vi "_DSF file channels to data.vi"(8 "error in (no error)":errorcluster, 10 "transfer":T7, 11 "configuration file cluster in":T1) -> (0 "error out":errorcluster, 2 "channels":T13[](array[typedef]), 3 "configuration file cluster out":T1)   [LabVIEW 2017, in "DSF Configuration API v1.0.0.lvlib"]
uses:
  DSF Configuration API v1.0.0.lvlib
  Controls/dsf configuration data/1.0.0/dsf settings.ctl
  Controls/dsf configuration data/1.0.0/dsf configuration data v1.0.0.lvlib
  Controls/dsf configuration data/1.0.0/dsf channel.ctl
  get item value by id/get channel value by id.vi
  get item value by id/get setting value by id.vi
  Controls/dsf configuration file/1.0.0/DSF Transfer.ctl
  File API/DSFConfig.lvlib
  Controls/dsf configuration file/1.0.0/DSF Channel.ctl
  Controls/dsf configuration file/1.0.0/dsf timing.ctl
  Controls/dsf configuration file/1.0.0/DSF Group.ctl
  Controls/dsf configuration file/1.0.0/DSF Plugin.ctl
  Controls/dsf configuration file/1.0.0/Version Info.ctl
  Controls/dsf configuration file/1.0.0/DSF Settings.ctl
  Controls/dsf configuration file/1.0.0/DSF Config.ctl
  Controls/dsf configuration file/1.0.0/DSF Channel Info.ctl
  Controls/dsf configuration file/1.0.0/DSF Settings Info.ctl
  Controls/dsf configuration file/1.0.0/DSF Transfer Info.ctl
  File API/DSF Plugin Info.ctl
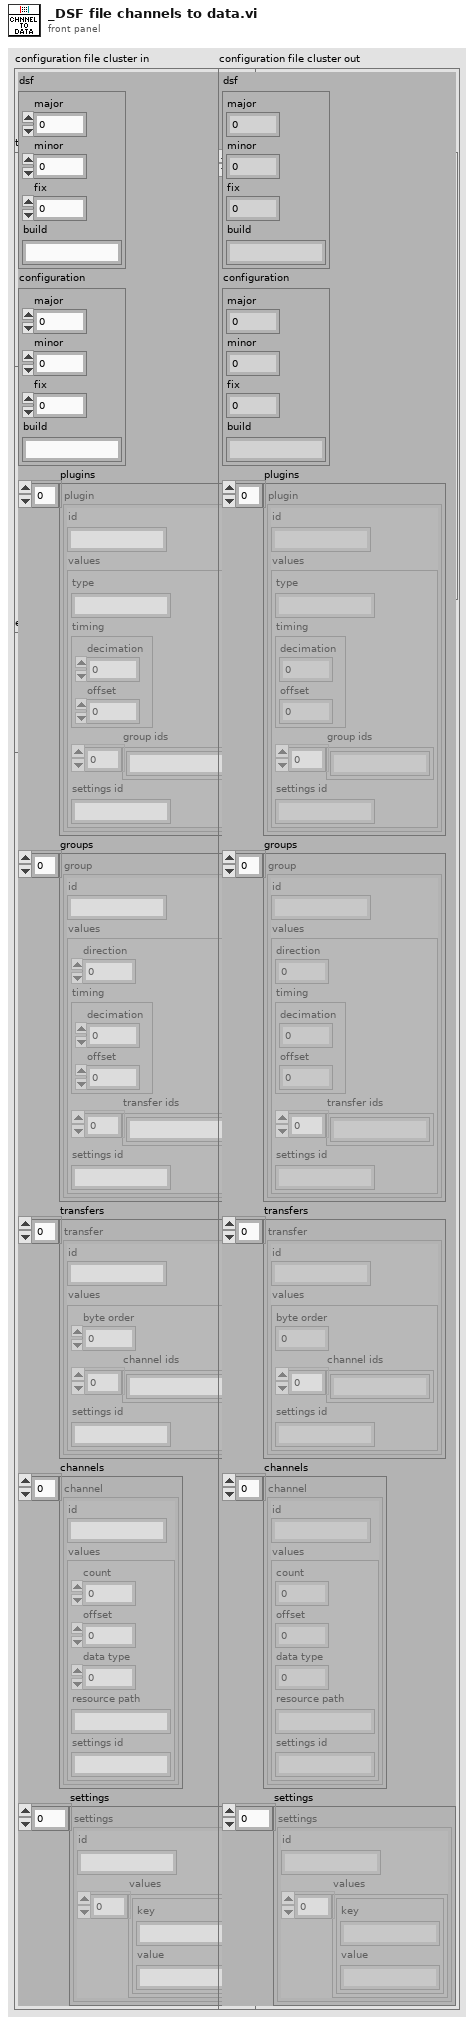
[diagram p1: front panel]
types:
  T1 = typedef "DSFConfig.lvlib/DSF Config.ctl" = cluster{"dsf":T2, "configuration":T2, "plugins":T3[], "groups":T6[], "transfers":T7[], "channels":T9[], "settings":T11[]}
  T2 = typedef "DSFConfig.lvlib/Version Info.ctl" = cluster{"major":u32, "minor":u32, "fix":u32, "build":string}
  T3 = typedef "DSFConfig.lvlib/DSF Plugin.ctl" = cluster{"id":string, "values":T4}
  T4 = typedef "DSFConfig.lvlib/DSF Plugin Info.ctl" = cluster{"type":string, "timing":T5, "group ids":string[], "settings id":string}
  T5 = typedef "DSFConfig.lvlib/dsf timing.ctl" = cluster{"decimation":i32, "offset":i32}
  T6 = typedef "DSFConfig.lvlib/DSF Group.ctl" = cluster{"id":string, "values":cluster{"direction":i32, "timing":T5, "transfer ids":string[], "settings id":string}}
  T7 = typedef "DSFConfig.lvlib/DSF Transfer.ctl" = cluster{"id":string, "values":T8}
  T8 = typedef "DSFConfig.lvlib/DSF Transfer Info.ctl" = cluster{"byte order":i32, "channel ids":string[], "settings id":string}
  T9 = typedef "DSFConfig.lvlib/DSF Channel.ctl" = cluster{"id":string, "values":T10}
  T10 = typedef "DSFConfig.lvlib/DSF Channel Info.ctl" = cluster{"count":i32, "offset":i32, "data type":i32, "resource path":string, "settings id":string}
  T11 = typedef "DSFConfig.lvlib/DSF Settings.ctl" = cluster{"id":string, "values":T12}
  T12 = typedef "DSFConfig.lvlib/DSF Settings Info.ctl" = cluster{"key":string, "value":string}[]
  T13 = typedef "dsf configuration data v1.0.0.lvlib/dsf channel.ctl" = cluster{"id":string, "values":cluster{"count":i32, "offset":i32, "data type":i32, "resource path":string, "settings":T14}}
  T14 = typedef "dsf configuration data v1.0.0.lvlib/dsf settings.ctl" = cluster{"id":string, "values":cluster{"key":string, "value":string}[]}
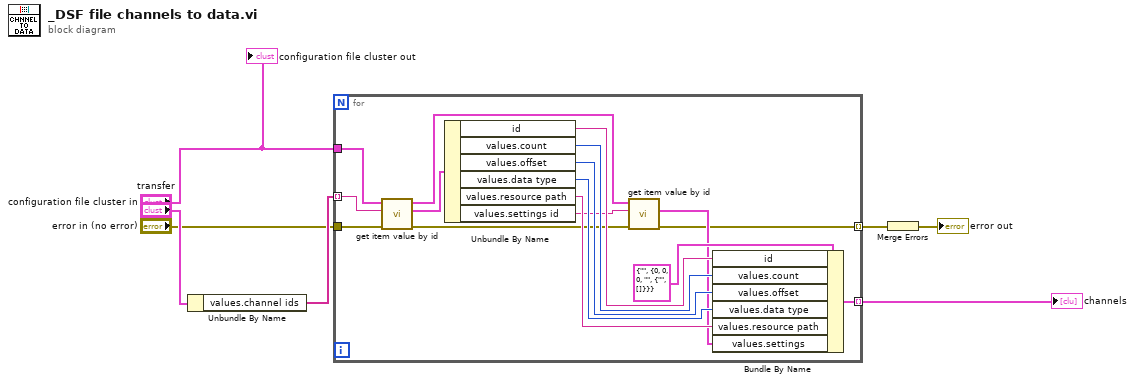
[diagram p0: block diagram]
diagram:
  n1 = Unbundle By Name("transfer") -> ("values.channel ids"=w7:string[])
  n2 = for {
    tunnel: "configuration file cluster in" -> [w23]
    tunnel: w7 -> [w22] mode=indexing
    tunnel: [w20] -> w1 mode=indexing
    tunnel: "error in (no error)" -> [w10]
    tunnel: [w8] -> w4 mode=indexing
    n3 = call-poly "get item value by id.vi"("error in (no error)"=w10, "id"=w22, "configuration file cluster in"=w23) -> ("error out"=w9:errorcluster, "channel"=w19:T9, "configuration file cluster out"=w13:T1)  [unwired: 5 in, 1 out]
    n4 = Unbundle By Name(w19) -> ("id"=w18:string, "values.count"=w17:i32, "values.offset"=w16:i32, "values.data type"=w15:i32, "values.resource path"=w14:string, "values.settings id"=w12:string)
    n5 = call-poly "get item value by id.vi"("error in (no error)"=w9, "id"=w12, "configuration file cluster in"=w13) -> ("error out"=w8:errorcluster, "settings"=w11:T11)  [unwired: 5 in, 2 out]
    n6 = Bundle By Name(cluster=T13 {"id"="", "values"={"count"=0, "offset"=0, "data type"=0, "resource path"="", "settings"={"id"="", "values"=[]}}} ("channel"), "id"=w18, "values.count"=w17, "values.offset"=w16, "values.data type"=w15, "values.resource path"=w14, "values.settings"=w11) -> (w20:T13)
  }
  "channels" <- w1
  n7 = Merge Errors(w4) -> (→"error out":errorcluster)
  "configuration file cluster out" <- "configuration file cluster in"
